vi "NGTS_DAQmx AI Read Data.vi"(8 "error  in":errorcluster, 11 "AI Tasks In":refnum<k21>) -> (0 "error out":errorcluster, 1 "Raw 1D Data out":dbl[](array[numeric]), 3 "AI Tasks Out":refnum<k21>)   [LabVIEW 2018]
uses:
  <vilib>/DAQmx/read.llb/DAQmx Read (Analog 1D Wfm NChan NSamp).vi
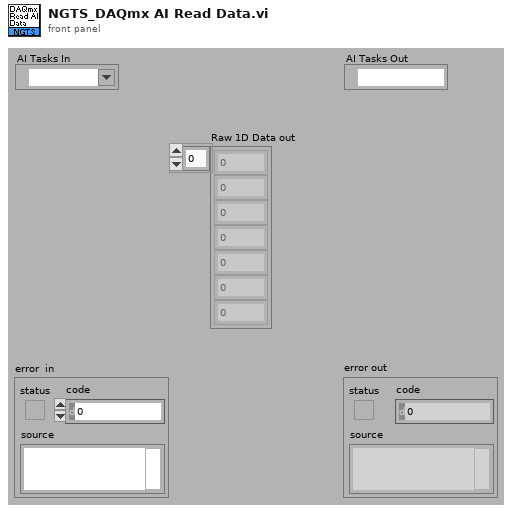
[diagram p1: front panel]
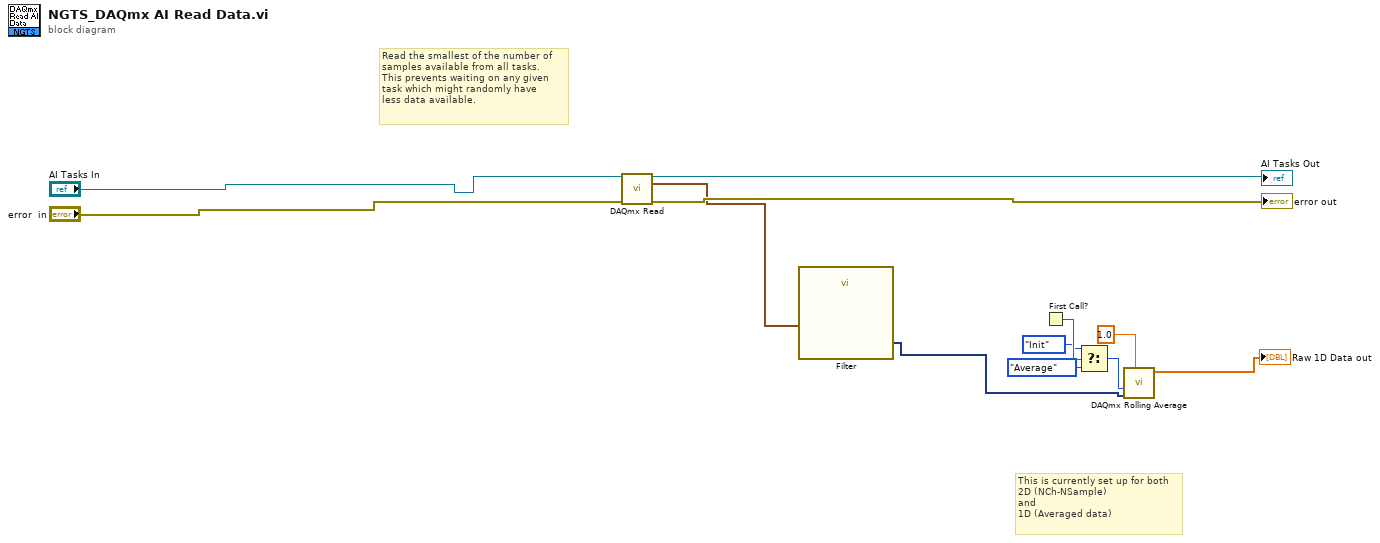
[diagram p0: block diagram]
diagram:
  # "Read the smallest of the number of\nsamples available from all tasks.\nThis prevents waiting on any given\ntask which might randomly have\nless data available."
  # "This is currently set up for both\n2D (NCh-NSample)\nand\n1D (Averaged data)"
  n1 = call-poly <vilib>:"DAQmx Read.vi"("task/channels in"="AI Tasks In", "error in"="error  in") -> ("task out"=→"AI Tasks Out":refnum<k21>, "data"=w11:waveform(dbl)[], "error out"=→"error out":errorcluster)  [unwired: 11 in]
  n2 = call "Filter"("Signal"=w11) -> ("Filtered Signal"=w10:dynamicdata)  [unwired: 9 in, 1 out]
  n3 = First Call?() -> (First Call?: T/F=w5:bool)
  n4 = Select(t=enum16{"Average", "Init"}."Init" ("Enum"), s=w5, f=enum16{"Average", "Init"}."Average") -> (s? t:f=w1:enum16{"Average", "Init"})
  n5 = call "DAQmx Rolling Average.vi"("Seconds to Average"=1.0, "Signal"=w10, "Action"=w1) -> ("Mean Array"=→"Raw 1D Data out":dbl[], "Sample Rate"=w9:dbl)  [unwired: 7 in]
